vi "database1查询.vi"(6 "时间2":string, 7 "error in (no error)":errorcluster, 8 "table":string, 9 "时间1":string, 10 "database":string="database1.mdb") -> (0 "error out":errorcluster, 2 "data":string[][](table), 3 "recordset data":variant[][](array[variant]))   [LabVIEW 2016, in "数据传输系统.lvlib"]
uses:
  <vilib>/Utility/sysdir.llb/System Directory Type.ctl
  <vilib>/addons/database/Connection.llb/DB Tools Open Connec (String).vi
  <vilib>/addons/database/Connection.llb/Conn Execute.vi
  <vilib>/addons/database/Recordset.llb/Rec Fetch Recordset Data (R).vi
  <vilib>/addons/database/Recordset.llb/Rec Destroy - Connection.vi
  <vilib>/addons/database/_DB Variant To Data/Database Variant To Data.xnode
  <vilib>/addons/database/NI_Database_API.lvlib
panel:
  out "SQL query":string
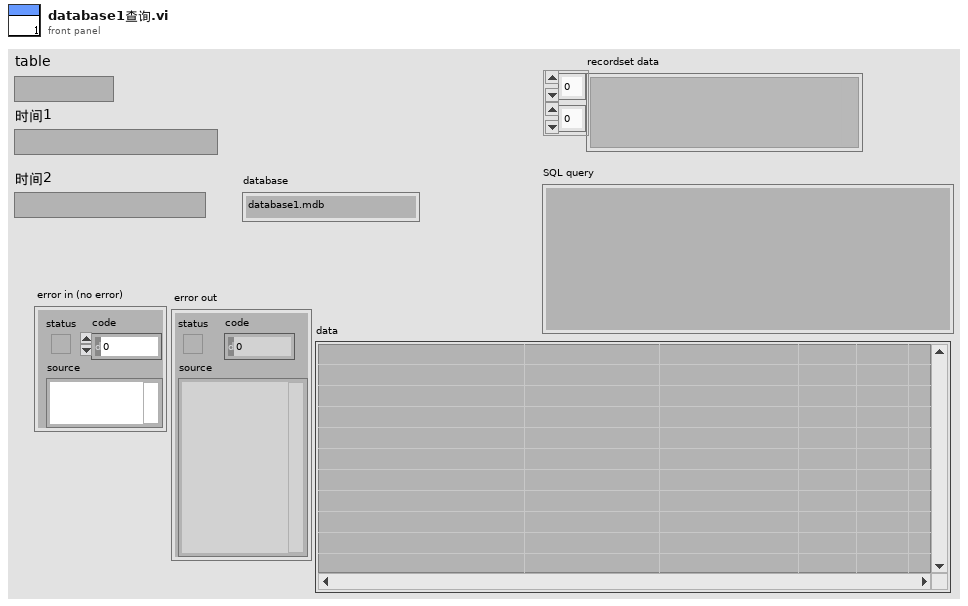
[diagram p1: front panel]
types:
  T1 = typedef "System Directory Type.ctl" = i32
  T2 = typedef "NI_Database_API.lvlib/Conn ObjectReference.ctl" = refnum<k1>
  T3 = typedef "NI_Database_API.lvlib/Rec ObjectReference.ctl" = refnum<k1>
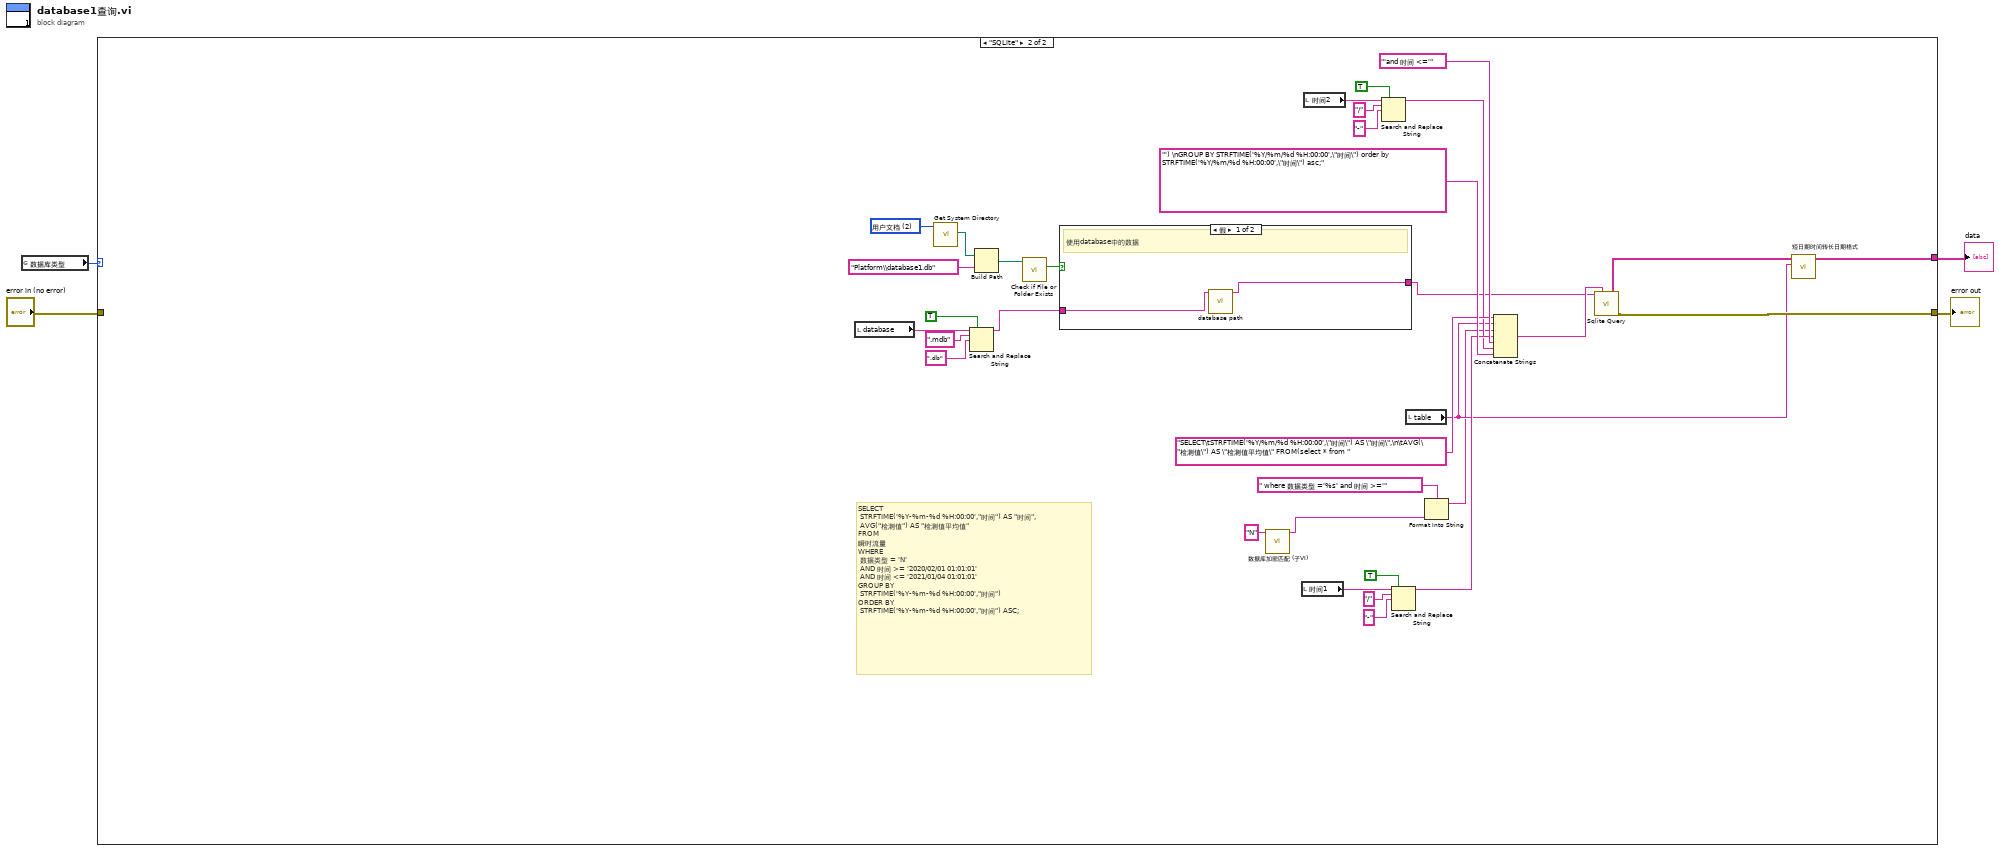
[diagram p0: block diagram]
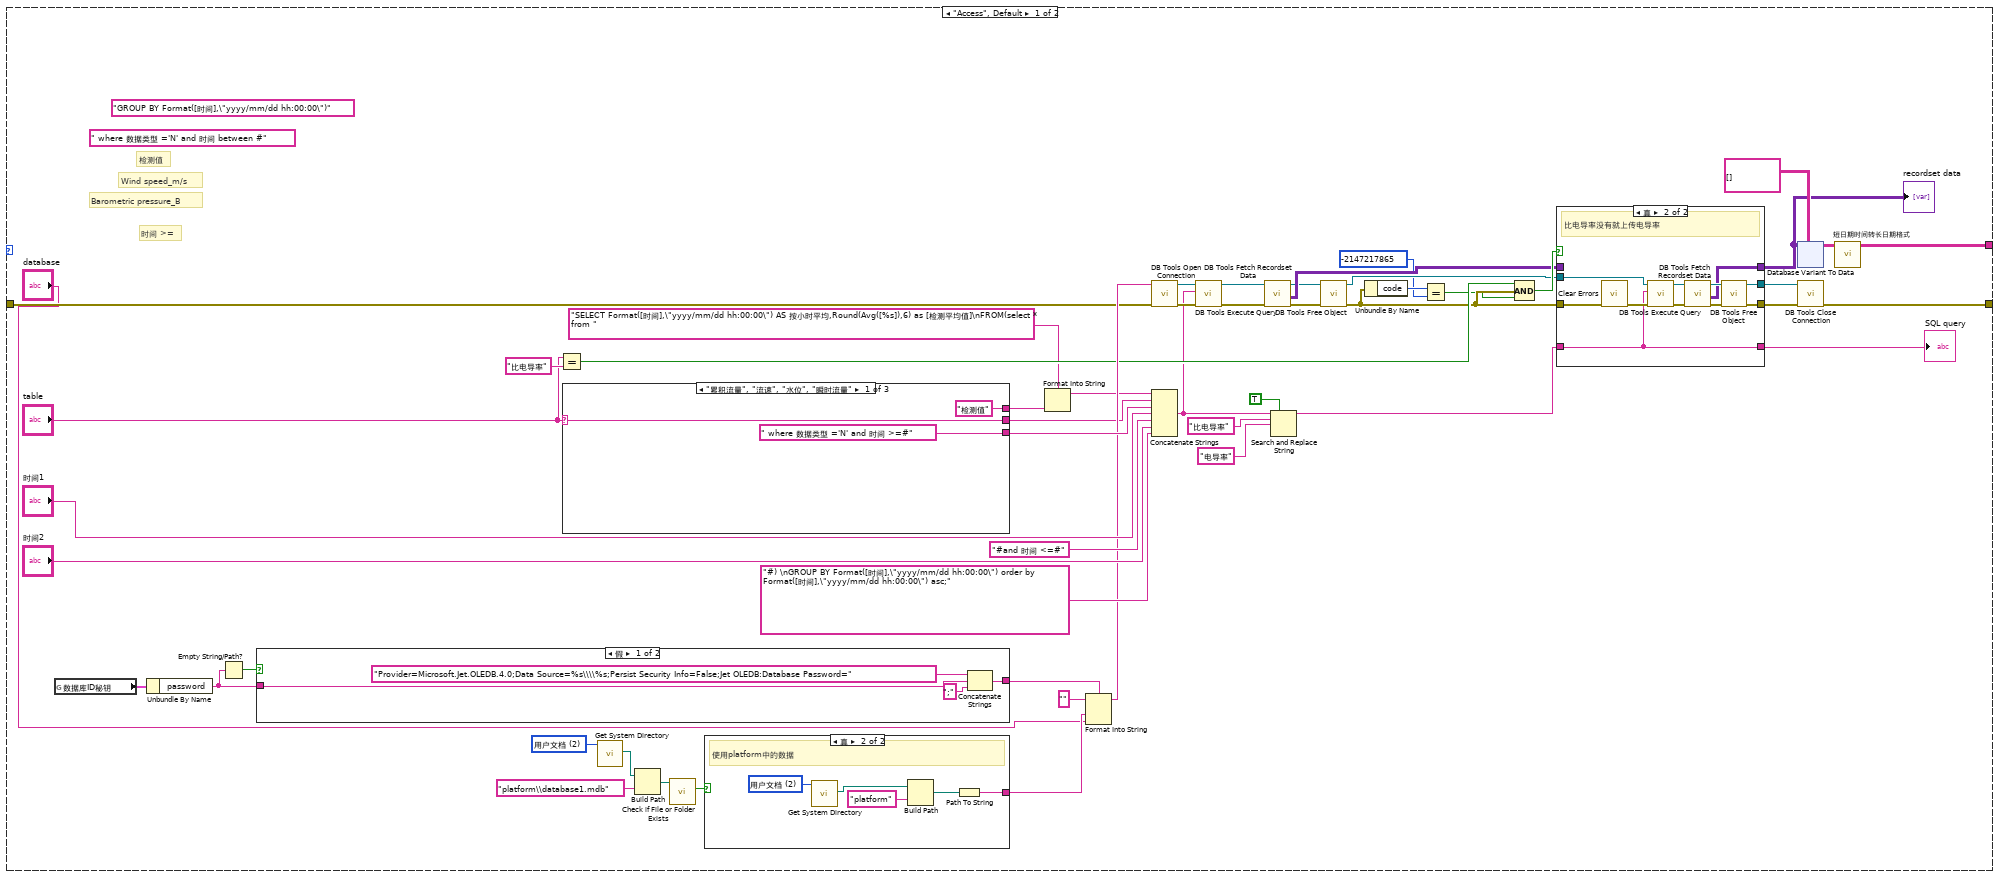
[diagram p2: hidden frame]
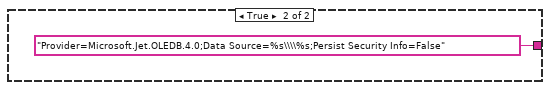
[diagram p3: hidden frame]
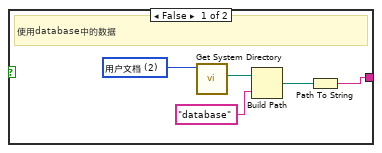
[diagram p5: hidden frame]
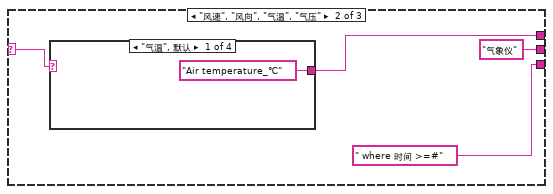
[diagram p6: hidden frame]
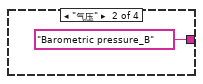
[diagram p7: hidden frame]
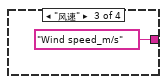
[diagram p8: hidden frame]
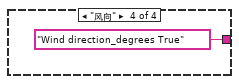
[diagram p9: hidden frame]
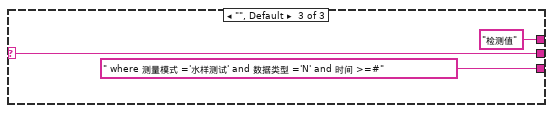
[diagram p10: hidden frame]
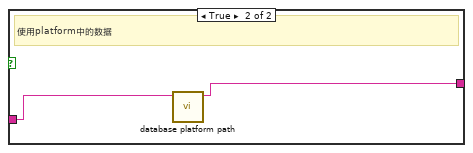
[diagram p11: hidden frame]
diagram:
  n1 = global read "断电保存全局.vi" "数据库类型"() -> (w3:enum16{"Access", "SQLite"})
  n2 = case shown="\"SQLite\"" w3 {
    tunnel: [w12 w154] -> w4
    tunnel: "error in (no error)" -> [w11 _]
    tunnel: [w6 w170] -> w1
    frame "Access", Default {
      (unwired) " where 数据类型 ='N' and 时间 between #"
      w47 = T1 2 items=["用户目录"=0, "用户桌面"=1, "用户文档"=2, "用户应用程序数据"=3, "用户设置"=4, "用户临时目录"=5, "公共文档"=6, "公共应用程序数据"=7, "公共设置"=8, "公共缓存"=13, "系统核心库"=9, "系统安装库"=10, "应用程序文件"=11, "启动盘根目录"=12] ("system directory type")
      (unwired) "GROUP BY Format([时间],\"yyyy/mm/dd hh:00:00\")"
      # "时间 >="
      # "Wind speed_m/s"
      # "检测值"
      # "Barometric pressure_B"
      n3 = global read "外部交互全局.vi" "数据库ID秘钥"() -> (w13:cluster{"userID":string, "password":string})
      n4 = Unbundle By Name(w13) -> ("password"=w15:string)
      n5 = Empty String/Path?(string/path=w15) -> (empty?=w16:bool)
      n6 = case shown="假" w16 {
        tunnel: [w101 "Provider=Microsoft.Jet.OLEDB.4.0;Data Source=%s\\\\%s;Persist Security Info=False" ("格式字符串")] -> w14
        tunnel: w15 -> [w104 _]
        frame False {
          n7 = Concatenate Strings("Provider=Microsoft.Jet.OLEDB.4.0;Data Source=%s\\\\%s;Persist Security Info=False;Jet OLEDB:Database Password=" ("格式字符串"), w104, ";" ("字符串")) -> (w101:string)
        }
        frame True {
        }
      }
      n8 = Equal?(x="table", y="比电导率") -> (x = y?=w36:bool)
      n9 = case shown="\"累积流量\", \"流速\", \"水位\", \"瞬时流量\"" "table" {
        selector: "table" -> [w132 w135 w143]
        tunnel: [" where 数据类型 ='N' and 时间 >=#" " where 时间 >=#" " where 测量模式 ='水样测试' and 数据类型 ='N' and 时间 >=#"] -> w50
        tunnel: ["检测值" w134 "检测值"] -> w20
        tunnel: [w132 "气象仪" w143] -> w18
        frame "累积流量", "流速", "水位", "瞬时流量" {
        }
        frame "风速", "风向", "气温", "气压" {
          n10 = case shown="\"气温\", 默认" w135 {
            tunnel: ["Air temperature_℃" "Barometric pressure_B" "Wind speed_m/s" "Wind direction_degrees True"] -> w134
            frame "气温", Default {
            }
            frame "气压" {
            }
            frame "风速" {
            }
            frame "风向" {
            }
          }
        }
        frame "", Default {
        }
      }
      n11 = call <vilib>:"Get System Directory.vi"("system directory type"=w47) -> ("system directory"=w48:path)  [unwired: 10 in]
      n12 = Build Path(base path=w48, name or relative path="platform\\database1.mdb" ("condition")) -> (appended path=w46:path)
      n13 = call <vilib>:"Check if File or Folder Exists.vi"("path"=w46) -> ("file or folder exists?"=w44:bool)  [unwired: 8 in, 2 out]
      n14 = case shown="真" w44 {
        tunnel: [w121 w126] -> w43
        frame False {
          w124 = T1 2 items=["用户目录"=0, "用户桌面"=1, "用户文档"=2, "用户应用程序数据"=3, "用户设置"=4, "用户临时目录"=5, "公共文档"=6, "公共应用程序数据"=7, "公共设置"=8, "公共缓存"=13, "系统核心库"=9, "系统安装库"=10, "应用程序文件"=11, "启动盘根目录"=12] ("system directory type")
          # "使用database中的数据"
          n15 = call <vilib>:"Get System Directory.vi"("system directory type"=w124) -> ("system directory"=w123:path)  [unwired: 10 in]
          n16 = Build Path(base path=w123, name or relative path="database" ("condition")) -> (appended path=w125:path)
          n17 = Path To String(path=w125) -> (string=w121:string)
        }
        frame True {
          w130 = T1 2 items=["用户目录"=0, "用户桌面"=1, "用户文档"=2, "用户应用程序数据"=3, "用户设置"=4, "用户临时目录"=5, "公共文档"=6, "公共应用程序数据"=7, "公共设置"=8, "公共缓存"=13, "系统核心库"=9, "系统安装库"=10, "应用程序文件"=11, "启动盘根目录"=12] ("system directory type")
          # "使用platform中的数据"
          n18 = call <vilib>:"Get System Directory.vi"("system directory type"=w130) -> ("system directory"=w129:path)  [unwired: 10 in]
          n19 = Build Path(base path=w129, name or relative path="platform" ("condition")) -> (appended path=w127:path)
          n20 = Path To String(path=w127) -> (string=w126:string)
        }
      }
      n21 = Format Into String(format string="SELECT Format([时间],\"yyyy/mm/dd hh:00:00\") AS 按小时平均,Round(Avg([%s]),6) as [检测平均值]\nFROM(select * from ", w20) -> (resulting string=w17:string)  [unwired: 2 in, 1 out]
      n22 = Format Into String(format string=w14, initial string="" ("初始字符串"), w43, "database") -> (resulting string=w42:string)  [unwired: 1 in, 1 out]
      n23 = call-poly <vilib>:"DB Tools Open Connection.vi"("error in (no error)"=w11, "connection information"=w42) -> ("error out"=w55:errorcluster, "connection reference"=w38:T2)  [unwired: 6 in]
      n24 = Concatenate Strings(w17, w18, w50, "时间1", "#and 时间 <=#", "时间2", "#) \nGROUP BY Format([时间],\"yyyy/mm/dd hh:00:00\") order by Format([时间],\"yyyy/mm/dd hh:00:00\") asc;" ("字符串")) -> (w27:string)
      n25 = call-poly <vilib>:"DB Tools Execute Query.vi"("error in (no error)"=w55, "SQL query"=w27, "connection reference"=w38) -> ("error out"=w34:errorcluster, "recordset reference"=w39:T3)  [unwired: 5 in]
      n26 = call-poly <vilib>:"DB Tools Fetch Recordset Data.vi"("error in (no error)"=w34, "recordset reference"=w39) -> ("error out"=w56:errorcluster, "recordset data"=w40:variant[][], "recordset reference out"=w35:T3)  [unwired: 3 in]
      n27 = Search and Replace String(replace all?=TRUE ("替换全部？(F)"), input string=w27, search string="比电导率" ("搜索字符串"), replace string="电导率" ("替换字符串(\"\")")) -> (result string=w24:string)  [unwired: 4 in, 3 out]
      n28 = call-poly <vilib>:"DB Tools Free Object.vi"("error in (no error)"=w56, "recordset reference"=w35) -> ("error out"=w29:errorcluster, "connection reference"=w33:T2)  [unwired: 8 in]
      n29 = Unbundle By Name(w29) -> ("code"=w31:i32)
      n30 = Equal?(x=w31, y=-2147217865 ("code")) -> (x = y?=w28:bool)
      n31 = Compound Arithmetic op=AND ("复合运算")(w36, w29, w28) -> (w41:bool)
      n32 = case shown="真" w41 {
        tunnel: w24 -> [w106 w110]
        tunnel: w33 -> [w107 w115]
        tunnel: [w107 w111] -> w32
        tunnel: [w109 w113] -> w7
        tunnel: w40 -> [w109 _]
        tunnel: w29 -> [w108 w120]
        tunnel: [w108 w112] -> w8
        tunnel: [w106 w110] -> w22
        frame False {
        }
        frame True {
          # "比电导率没有就上传电导率"
          n33 = call <vilib>:"Clear Errors.vi"("error in (no error)"=w120) -> ("error out"=w114:errorcluster)  [unwired: 5 in, 1 out]
          n34 = call-poly <vilib>:"DB Tools Execute Query.vi"("error in (no error)"=w114, "SQL query"=w110, "connection reference"=w115) -> ("error out"=w116:errorcluster, "recordset reference"=w118:T3)  [unwired: 5 in]
          n35 = call-poly <vilib>:"DB Tools Fetch Recordset Data.vi"("error in (no error)"=w116, "recordset reference"=w118) -> ("error out"=w119:errorcluster, "recordset data"=w113:variant[][], "recordset reference out"=w117:T3)  [unwired: 3 in]
          n36 = call-poly <vilib>:"DB Tools Free Object.vi"("error in (no error)"=w119, "recordset reference"=w117) -> ("error out"=w112:errorcluster, "connection reference"=w111:T2)  [unwired: 8 in]
        }
      }
      "SQL query" <- w22
      "recordset data" <- w7
      n37 = xnode "Database Variant To Data"("database variant"=w7, "type"=string[][] []) -> ("data"=w9:string[][])  [unwired: 1 in, 1 out]
      n38 = call <vilib>:"DB Tools Close Connection.vi"("error in (no error)"=w8, "connection reference"=w32) -> ("error out"=w12:errorcluster)  [unwired: 5 in]
      n39 = call "短日期时间转长日期格式.vi"("data"=w9) -> ("输出数组"=w6:string[][])  [unwired: 10 in]
    }
    frame "SQLite" {
      w174 = T1 2 items=["用户目录"=0, "用户桌面"=1, "用户文档"=2, "用户应用程序数据"=3, "用户设置"=4, "用户临时目录"=5, "公共文档"=6, "公共应用程序数据"=7, "公共设置"=8, "公共缓存"=13, "系统核心库"=9, "系统安装库"=10, "应用程序文件"=11, "启动盘根目录"=12] ("system directory type")
      # "SELECT\n\tSTRFTIME('%Y-%m-%d %H:00:00',\"时间\") AS \"时间\",\n\tAVG(\"检测值\") AS \"检测值平均值\"\nFROM\n瞬时流量 \nWHERE\n\t数据类型 = 'N' \n\tAND 时间 >= '2020/02/01 01:01:01' \n\tAND 时间 <= '2021/01/04 01:01:01' \nGROUP BY\n\tSTRFTIME('%Y-%m-%d %H:00:00',\"时间\")\nORDER BY\n\tSTRFTIME('%Y-%m-%d %H:00:00',\"时间\") ASC;"
      n40 = local read "database"() -> (w155:string)
      n41 = call <vilib>:"Get System Directory.vi"("system directory type"=w174) -> ("system directory"=w173:path)  [unwired: 10 in]
      n42 = Search and Replace String(replace all?=TRUE ("替换全部？(F)"), input string=w155, search string=".mdb" ("搜索字符串"), replace string=".db" ("替换字符串(\"\")")) -> (result string=w146:string)  [unwired: 4 in, 3 out]
      n43 = Build Path(base path=w173, name or relative path="Platform\\database1.db" ("condition")) -> (appended path=w175:path)
      n44 = call <vilib>:"Check if File or Folder Exists.vi"("path"=w175) -> ("file or folder exists?"=w177:bool)  [unwired: 8 in, 2 out]
      n45 = case shown="假" w177 {
        tunnel: [w178 w180] -> w145
        tunnel: w146 -> [w179 w181]
        frame False {
          # "使用database中的数据"
          n46 = call "database path.vi"("database"=w179) -> ("Path out"=w178:string)  [unwired: 9 in, 1 out]
        }
        frame True {
          # "使用platform中的数据"
          n47 = call "database platform path.vi"("database"=w181) -> ("Path out"=w180:string)  [unwired: 10 in]
        }
      }
      n48 = call "数据库加密匹配 (子VI).vi"("输入参数"="N") -> ("Encoded String"=w148:string)  [unwired: 10 in]
      n49 = local read "时间1"() -> (w162:string)
      n50 = local read "时间2"() -> (w160:string)
      n51 = Search and Replace String(replace all?=TRUE ("替换全部？(F)"), input string=w160, search string="/" ("搜索字符串"), replace string="-" ("替换字符串(\"\")")) -> (result string=w159:string)  [unwired: 4 in, 3 out]
      n52 = Search and Replace String(replace all?=TRUE ("替换全部？(F)"), input string=w162, search string="/" ("搜索字符串"), replace string="-" ("替换字符串(\"\")")) -> (result string=w161:string)  [unwired: 4 in, 3 out]
      n53 = local read "table"() -> (w152:string)
      n54 = Format Into String(format string=" where 数据类型 ='%s' and 时间 >='", w148) -> (resulting string=w150:string)  [unwired: 2 in, 1 out]
      n55 = Concatenate Strings("SELECT\tSTRFTIME('%Y/%m/%d %H:00:00',\"时间\") AS \"时间\",\n\tAVG(\"检测值\") AS \"检测值平均值\" FROM(select * from ", w152, w150, w161, "'and 时间 <='", w159, "') \nGROUP BY STRFTIME('%Y/%m/%d %H:00:00',\"时间\") order by STRFTIME('%Y/%m/%d %H:00:00',\"时间\") asc;" ("字符串")) -> (w147:string)
      n56 = call "Sqlite Query.vi"("DB Path"=w145, "SQL Query"=w147) -> ("Results"=w153:string[][], "error out"=w154:errorcluster)  [unwired: 11 in, 1 out]
      n57 = call "短日期时间转长日期格式.vi"("table输入"=w152, "data"=w153) -> ("输出数组"=w170:string[][])  [unwired: 9 in]
    }
  }
  "error out" <- w4
  "data" <- w1
